vi "to string.vi"(8 "error in":errorcluster, 11 "TDMS datalogger configuration in":refnum<class "TDMS datalogger configuration.lvclass">) -> (0 "error out":errorcluster, 1 "data":string, 2 "version":string, 3 "TDMS datalogger configuration out":refnum<class "TDMS datalogger configuration.lvclass">)   [LabVIEW 2013, in "TDMS datalogger configuration.lvclass"]
doc: "Provides an interface for saving a module configuration to a file or other serialized data source. It is recommended that all children of this class store data in two sets--data required for its own initialization, and any data required for parent initialization--and that each implementation uses the <b>Call Parent Method</b> primitive to serialize parent information."
uses:
  TDMS datalogger configuration.lvclass
  <vilib>/NI/Tag Bus Module Framework/module configuration/TBM module configuration.lvclass
  TDMS datalogger configuration.lvclass/TDMS datalogger configuration.ctl
  current version.vi
  <vilib>/NI/Tag Bus Module Framework/root configuration/TBM configuration.lvclass
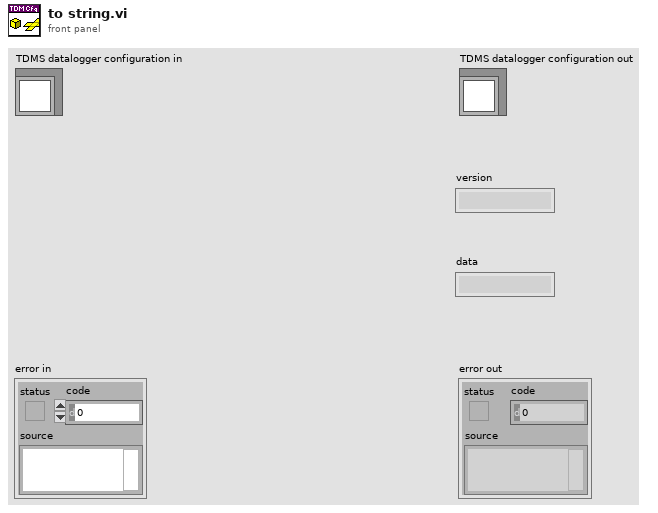
[diagram p1: front panel]
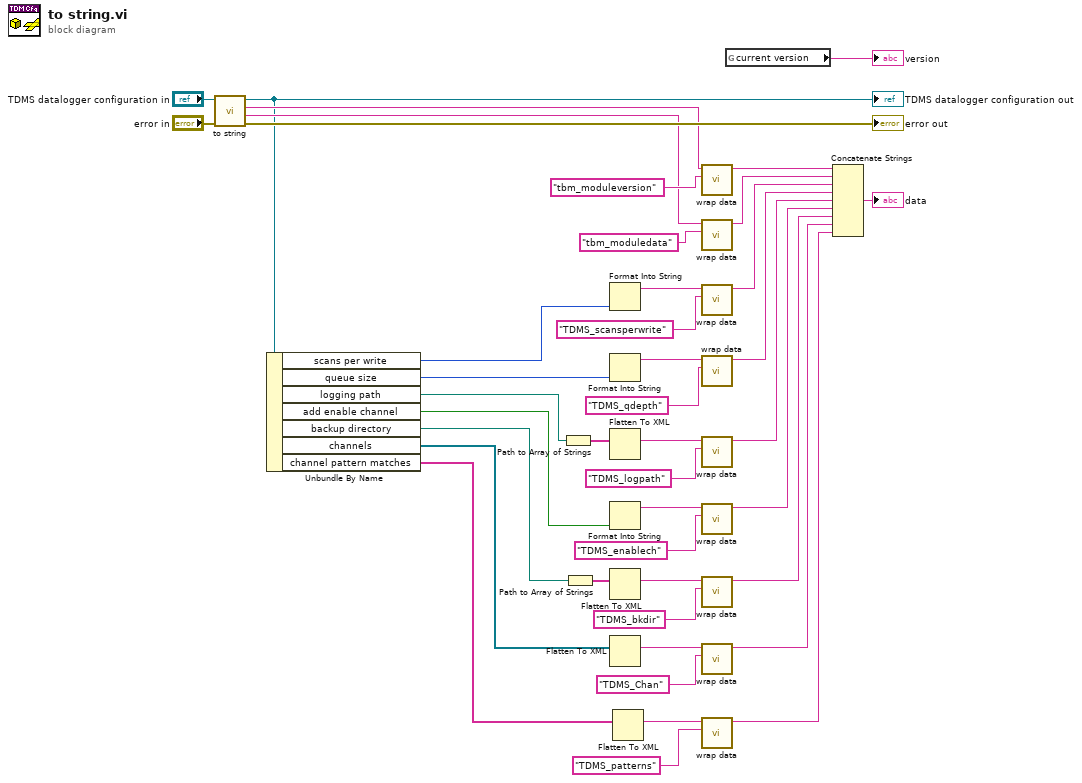
[diagram p0: block diagram]
diagram:
  n1 = call-parent "to string.vi"("error in"="error in", "module configuration in"="TDMS datalogger configuration in") -> ("error out"=→"error out":errorcluster, "data"=w35:string, "version"=w36:string, "module configuration out"=w31:refnum<class "TDMS datalogger configuration.lvclass">)  [unwired: 6 in]
  "TDMS datalogger configuration out" <- w31
  n2 = Unbundle By Name(w31) -> ("scans per write"=w23:i32, "queue size"=w24:i32, "logging path"=w27:path, "add enable channel"=w25:bool, "backup directory"=w29:path, "channels"=w30:refnum<class "TBM channel.lvclass">[], "channel pattern matches"=w4:string[])
  n3 = Path to Array of Strings(0:w27) -> (2:w26:string[])  [unwired: 1 out]
  n4 = Path to Array of Strings(0:w29) -> (2:w28:string[])  [unwired: 1 out]
  n5 = Format Into String(w23) -> (resulting string=w22:string)  [unwired: 3 in, 1 out]
  n6 = Format Into String(w24) -> (resulting string=w20:string)  [unwired: 3 in, 1 out]
  n7 = Flatten To XML(anything=w26) -> (xml string=w18:string)
  n8 = Format Into String(w25) -> (resulting string=w17:string)  [unwired: 3 in, 1 out]
  n9 = Flatten To XML(anything=w28) -> (xml string=w16:string)
  n10 = Flatten To XML(anything=w30) -> (xml string=w15:string)
  n11 = Flatten To XML(anything=w4) -> (xml string=w3:string)
  n12 = call <vilib>:"wrap data.vi"("identifier"="tbm_moduleversion" ("additional identifier"), "data to wrap"=w36) -> ("wrapped data"=w34:string)  [unwired: 9 in]
  n13 = call <vilib>:"wrap data.vi"("identifier"="tbm_moduledata" ("additional identifier"), "data to wrap"=w35) -> ("wrapped data"=w32:string)  [unwired: 9 in]
  n14 = call <vilib>:"wrap data.vi"("identifier"="TDMS_scansperwrite" ("additional identifier"), "data to wrap"=w22) -> ("wrapped data"=w21:string)  [unwired: 9 in]
  n15 = call <vilib>:"wrap data.vi"("identifier"="TDMS_qdepth" ("additional identifier"), "data to wrap"=w20) -> ("wrapped data"=w19:string)  [unwired: 9 in]
  n16 = call <vilib>:"wrap data.vi"("identifier"="TDMS_logpath" ("additional identifier"), "data to wrap"=w18) -> ("wrapped data"=w14:string)  [unwired: 9 in]
  n17 = call <vilib>:"wrap data.vi"("identifier"="TDMS_enablech" ("additional identifier"), "data to wrap"=w17) -> ("wrapped data"=w13:string)  [unwired: 9 in]
  n18 = call <vilib>:"wrap data.vi"("identifier"="TDMS_bkdir" ("additional identifier"), "data to wrap"=w16) -> ("wrapped data"=w12:string)  [unwired: 9 in]
  n19 = call <vilib>:"wrap data.vi"("identifier"="TDMS_Chan" ("additional identifier"), "data to wrap"=w15) -> ("wrapped data"=w11:string)  [unwired: 9 in]
  n20 = call <vilib>:"wrap data.vi"("identifier"="TDMS_patterns", "data to wrap"=w3) -> ("wrapped data"=w1:string)  [unwired: 9 in]
  n21 = global read "current version.vi" "current version"() -> (→"version":string)
  n22 = Concatenate Strings(w34, w32, w21, w19, w14, w13, w12, w11, w1) -> (→"data":string)
